vi "process_network.vi"(6 "Micron config":T12, 8 "Reset":bool, 9 "Goal position in":sgl[][](array[numeric]), 11 "Parameters":T1={"Stimulus"={"Type"=enum."Off", "Phase"=0.0, "Amplitude"=[], "Injection point"=enum."Total pose", "Closed loop"=FALSE, "Offset"=[], "Tip -> world"=FALSE, "Frequency"=0.0, "Length"=0.0}, "Goal Filter A"={"Speedup max"=0.0, "Speedup thresh"=0.0, "Speedup nonlin"=0.0, "Filters"=[]}, "Mode controls"={"Hold"=FALSE, "Cancellation"=FALSE, "Goal filter"=FALSE, "Trigger"=FALSE}, "Manipulator type"=enum."Current piezo", "Manipulator calibration"={"Tool offsets"=[[0.0, 0.0, 36200.0]], "Handle light calibration"=[], "Base pivots"=[], "Output pivots"=[], "Length center"=0.0, "Workspace height"=[], "Workspace diameter"=[0.0, 0.0, 36200.0], "Stack travel"=400.0, "Saturation pos"=375.0, "Inverse filters"=[], "Strut length"=0.0}, "Network"={"Remote Host"="", "Send Status"=FALSE, "Send Port"=0, "Recv Commands"=FALSE, "Recv Port"=0}, "Goal Filter B"={"Speedup max"=0.0, "Speedup thresh"=0.0, "Speedup nonlin"=0.0, "Filters"=[]}, "Cancellation"={"KP"={"XY"=0.0, "Rxy"=0.0, "Z"=0.0, "Rz"=0.0}, "KI"=0.0, "KD"={"XY"=0.0, "Rxy"=0.0, "Z"=0.0, "Rz"=0.0}, "Max vel"=20.0, "Max acc"=0.001, "Int error limit"=3.0, "RCM gain"=0.0, "Bypass"=FALSE, "Degraded gain"=0.0}, "Transition time"=0.0, "Estimation"={"Link"={"Measure noise"=[], "Process noise"=[], "Alt process noise"=[], "Alt turnoff cycles"=20, "Innovation limit"=[], "Residue threshold"=0.0, "Enable"=FALSE}, "Handle"={"Measure noise"=[], "Process noise"=[], "State limits"=[], "Innovation limit"=[], "Prediction Lookahead"=0.0, "Enable"=FALSE}}} {"Transition time" format="%_3f"; "Cancellation"."Degraded gain" min=0 max=1 step=0.1 format="%#_3p"; "Cancellation"."RCM gain" min=0 max=1 step=0.1 format="%#_3p"; "Cancellation"."KD"."Rz" min=-1 max=1 step=0.01 format="%#_3p"; "Cancellation"."KD"."Rxy" min=-1 max=1 step=0.01 format="%#_3p"; "Cancellation"."KD"."Z" min=-1 max=1 step=0.01 format="%#_3p"; "Cancellation"."KD"."XY" min=-1 max=1 step=0.01 format="%#_3p"; "Cancellation"."KI" min=0 max=1 step=0.01 format="%#_3p"; "Cancellation"."KP"."Rz" min=-1 max=1 step=0.01 format="%#_3p"; "Cancellation"."KP"."Rxy" min=-1 max=1 step=0.01 format="%#_3p"; "Cancellation"."KP"."Z" min=-1 max=1 step=0.01 format="%#_3p"; "Cancellation"."KP"."XY" min=-1 max=1 step=0.01 format="%#_3p"; "Cancellation"."Max acc" format="%#_3p"; "Goal Filter B"."Filters"."V limit range" format="%_3p"; "Goal Filter B"."Filters"."V limit" format="%_3p"; "Goal Filter B"."Filters"."Upper Q" format="%_3f"; "Goal Filter B"."Filters"."Upper Fc" format="%_3p"; "Goal Filter B"."Filters"."Lower Q" format="%_3f"; "Goal Filter B"."Filters"."Scale factor" format="%_3f"; "Goal Filter B"."Filters"."Lower Fc" format="%_3p"; "Goal Filter B"."Speedup nonlin" format="%_3p"; "Goal Filter B"."Speedup thresh" format="%_3p"; "Goal Filter B"."Speedup max" format="%_3p"; "Manipulator calibration"."Strut length" format="%#_4p"; "Manipulator calibration"."Saturation pos" format="%#.1f"; "Manipulator calibration"."Stack travel" format="%#.1f"; "Manipulator calibration"."Length center" format="%#_4p"; "Manipulator calibration"."Output pivots" format="%#_6f"; "Manipulator calibration"."Base pivots" format="%#_6f"; "Manipulator calibration"."Handle light calibration" format="%#.1f"; "Goal Filter A"."Filters"."V limit range" format="%_3p"; "Goal Filter A"."Filters"."V limit" format="%_3p"; "Goal Filter A"."Filters"."Upper Q" format="%_3f"; "Goal Filter A"."Filters"."Upper Fc" format="%_3p"; "Goal Filter A"."Filters"."Lower Q" format="%_3f"; "Goal Filter A"."Filters"."Scale factor" format="%_3f"; "Goal Filter A"."Filters"."Lower Fc" format="%_3p"; "Goal Filter A"."Speedup nonlin" format="%_3p"; "Goal Filter A"."Speedup thresh" format="%_3p"; "Goal Filter A"."Speedup max" format="%_3p"; "Stimulus"."Length" min=0.0 max=100.0 step=100.0 format="%#_4p"; "Stimulus"."Frequency" min=0.0 step=100.0 format="%#_4g"; "Stimulus"."Offset" format="%#_3p"; "Stimulus"."Amplitude" format="%#_3p"; "Stimulus"."Phase" min=-180.0 max=360.0 step=100.0 format="%#.2f"}) -> (5 "Goal position out":sgl[][](array[numeric]))   [LabVIEW 2014]
uses:
  initialization/micron_config.ctl
  manipulator/squiggle/Host/i2c_interface.ctl
  manipulator/squiggle/Host/fpga_reference.ctl
  testing/Micron params.ctl
  testing/stimulus.ctl
  testing/injection_point.ctl
  goal_loop_parms.ctl
  testing/mode_conrols.ctl
  testing/manipulator_cal.ctl
  asap/labview/testing/probe_calibration.ctl
  host/network_params.ctl
  cancellation/sq_control_params.ctl
  cancellation/decoupled_gain.ctl
  cancellation/estimation_controls.ctl
  <vilib>/DAQmx/write.llb/DAQmx Write (Digital Bool 1Line 1Point).vi
panel:
  out "Network command":sgl[](array[numeric])
  # "Local variables:"
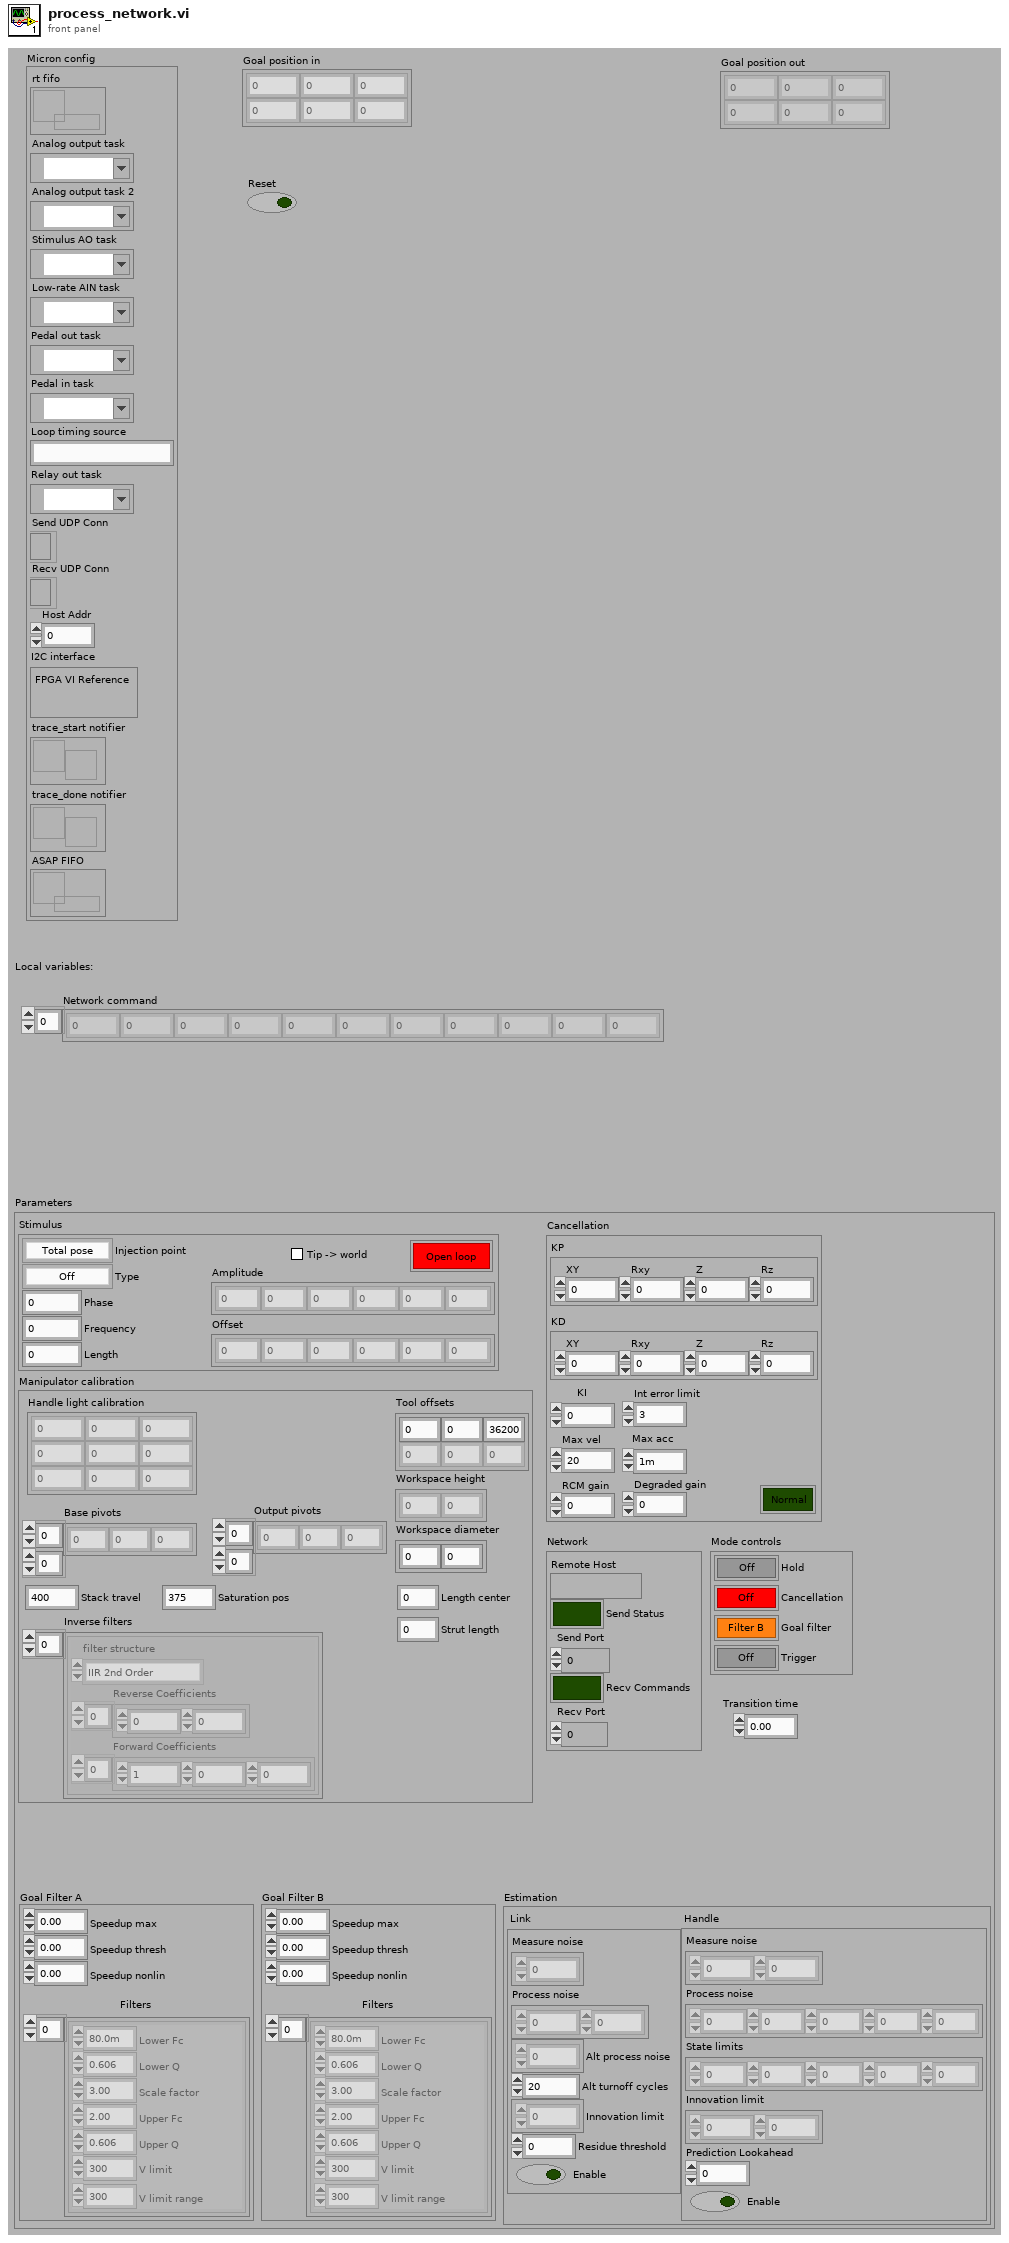
[diagram p1: front panel]
types:
  T1 = typedef "Micron params.ctl" = cluster{"Stimulus":T2, "Goal Filter A":T4, "Mode controls":T5, "Manipulator type":enum16{"Current piezo", "Voltage piezo"}, "Manipulator calibration":T6, "Network":T8, "Goal Filter B":T4, "Cancellation":T9, "Transition time":sgl, "Estimation":T11}
  T2 = typedef "stimulus.ctl" = cluster{"Type":enum16{"Off", "Step", "Sine", "Triangle", "Arbitrary"}, "Phase":dbl, "Amplitude":sgl[], "Injection point":T3, "Closed loop":bool, "Offset":sgl[], "Tip -> world":bool, "Frequency":dbl, "Length":dbl}
  T3 = typedef "injection_point.ctl" = enum16{"Total pose", "V limiter", "Goal ", "Link position", "KF link position", "Inverse kin", "Link goal", "Link error", "Controller", "Output", "Drive", "Light"}
  T4 = typedef "goal_loop_parms.ctl" = cluster{"Speedup max":sgl, "Speedup thresh":sgl, "Speedup nonlin":sgl, "Filters":cluster{"Lower Fc":sgl, "Lower Q":sgl, "Scale factor":sgl, "Upper Fc":sgl, "Upper Q":sgl, "V limit":sgl, "V limit range":sgl}[]}
  T5 = typedef "mode_conrols.ctl" = cluster{"Hold":bool, "Cancellation":bool, "Goal filter":bool, "Trigger":bool}
  T6 = typedef "manipulator_cal.ctl" = cluster{"Tool offsets":sgl[][], "Handle light calibration":T7, "Base pivots":sgl[][], "Output pivots":sgl[][], "Length center":sgl, "Workspace height":sgl[], "Workspace diameter":sgl[], "Stack travel":sgl, "Saturation pos":sgl, "Inverse filters":cluster{"filter structure":enum32{"IIR 2nd Order", "IIR 4th Order"}, "Reverse Coefficients":dbl[], "Forward Coefficients":dbl[]}[], "Strut length":sgl}
  T7 = typedef "probe_calibration.ctl" = sgl[][]
  T8 = typedef "network_params.ctl" = cluster{"Remote Host":string, "Send Status":bool, "Send Port":u16, "Recv Commands":bool, "Recv Port":u16}
  T9 = typedef "sq_control_params.ctl" = cluster{"KP":T10, "KI":sgl, "KD":T10, "Max vel":sgl, "Max acc":sgl, "Int error limit":sgl, "RCM gain":sgl, "Bypass":bool, "Degraded gain":sgl}
  T10 = typedef "decoupled_gain.ctl" = cluster{"XY":sgl, "Rxy":sgl, "Z":sgl, "Rz":sgl}
  T11 = typedef "estimation_controls.ctl" = cluster{"Link":cluster{"Measure noise":dbl[], "Process noise":dbl[], "Alt process noise":dbl[], "Alt turnoff cycles":i32, "Innovation limit":dbl[], "Residue threshold":dbl, "Enable":bool}, "Handle":cluster{"Measure noise":dbl[], "Process noise":dbl[], "State limits":dbl[], "Innovation limit":dbl[], "Prediction Lookahead":sgl, "Enable":bool}}
  T12 = typedef "micron_config.ctl" = cluster{"rt fifo":refnum<k33>, "Analog output task":refnum<k21>, "Analog output task 2":refnum<k21>, "Stimulus AO task":refnum<k21>, "Low-rate AIN task":refnum<k21>, "Pedal out task":refnum<k21>, "Pedal in task":refnum<k21>, "Loop timing source":string, "Relay out task":refnum<k21>, "Send UDP Conn":refnum<k16>, "Recv UDP Conn":refnum<k16>, "Host Addr":u32, "I2C interface":T13, "trace_start notifier":refnum<notifier>, "trace_done notifier":refnum<notifier>, "ASAP FIFO":refnum<k33>}
  T13 = typedef "i2c_interface.ctl" = cluster{"FPGA VI Reference":T14}
  T14 = typedef "fpga_reference.ctl" = refnum<k20>
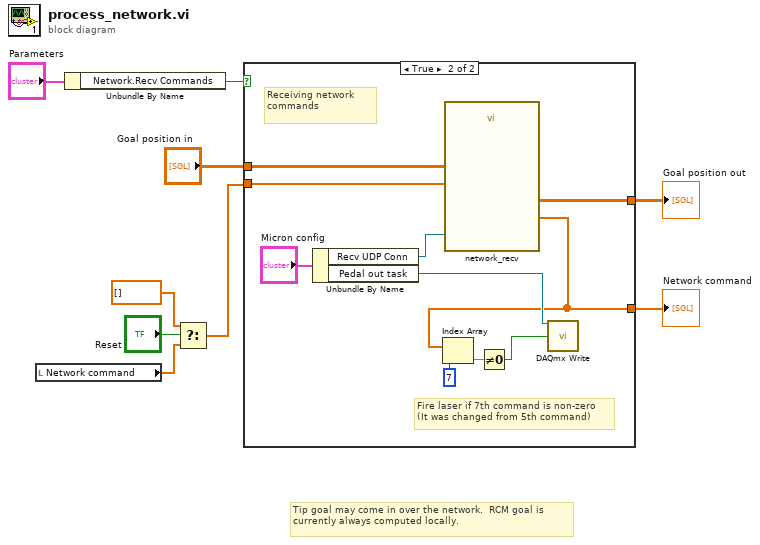
[diagram p0: block diagram]
diagram:
  # "Tip goal may come in over the network.  RCM goal is currently always computed locally."
  n1 = local read "Network command"() -> (w4:sgl[])
  n2 = Unbundle By Name("Parameters") -> ("Network.Recv Commands"=w8:bool)
  n3 = Select(t=sgl[] [] ("Network command"), s="Reset", f=w4) -> (s? t:f=w3:sgl[])
  n4 = case shown="True" w8 {
    tunnel: "Goal position in" -> [w11 w19]
    tunnel: [w11 w21] -> w1
    tunnel: w3 -> [w10 w20]
    tunnel: [w10 w12] -> w7
    frame False {
      # "Normal standalone operation"
    }
    frame True {
      # "Receiving network commands"
      # "Fire laser if 7th command is non-zero\n(It was changed from 5th command)"
      n5 = Unbundle By Name("Micron config") -> ("Recv UDP Conn"=w14:refnum<k16>, "Pedal out task"=w18:refnum<k21>)
      n6 = call "network_recv.vi"("Network In"=w20, "Goal position in"=w19, "Recv UDP Conn"=w14) -> ("Network Out"=w12:sgl[], "Goal position out"=w21:sgl[][])  [unwired: 7 in]
      n7 = Index Array(array=w12, index=7 ("t")) -> (element=w15:sgl)
      n8 = Not Equal To 0?(x=w15) -> (x != 0?=w16:bool)
      n9 = call-poly <vilib>:"DAQmx Write.vi"("task/channels in"=w18, "data"=w16) -> ()  [unwired: 2 in, 12 out]
    }
  }
  "Goal position out" <- w1
  "Network command" <- w7
